vi "_FPGA Check Turbo.vi"(4 "error in":errorcluster, 6 "CheckNow (F)":bool) -> (0 "error out":errorcluster, 2 "SpeedOK":bool)   [LabVIEW 2012]
uses:
  Type/_Pump Parameter.ctl
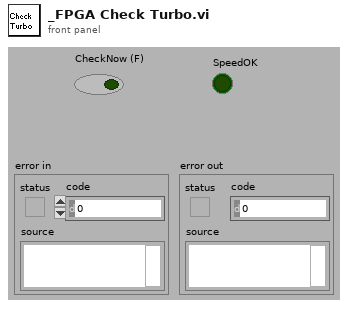
[diagram p1: front panel]
types:
  T1 = typedef "_Pump Parameter.ctl" = enum16{"Turn Pump Motor On", "Turn Pump Motor Off", "Read Pump Oil Deficiency", "Read Rotation Switch Point Attained", "Read Ele. Drive Over Temperature", "Read Pump Over Temperature", "Read Set Rotation Speed Attained", "Read Turbopump Accelerates", "Read Actual Rotation Speed in Hz", "Read Motor Current in A", "Read Operating Hours in h", "Read Motor Voltage in V", "Read Motor Power in W", "Set Rotation Speed Switchpoint in %", "Clear Error", "Read Error Code", "Read Bearing Temperature", "Read Hardware Version", "Read Firmware Version", "Read Operating Hours (Drive)", "Read Rotational Speed (rpm)", "Read Power Stage Temperature", "Read Electronics Temperature", "Read Upper Pump Temperature", "Read Motor Temperature", "Read Error Code History, 1", "Read Error Code History, 2", "Read Error Code History, 3", "Read Error Code History, 4", "Read Error Code History, 5", "Read Error Code History, 6", "Read Error Code History, 7", "Read Error Code History, 8", "Read Error Code History, 9", "Read Error Code History, 10"}
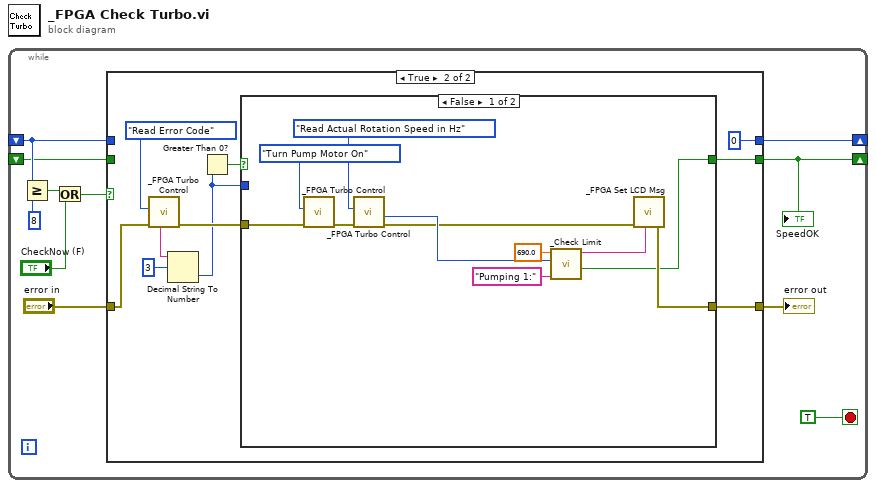
[diagram p0: block diagram]
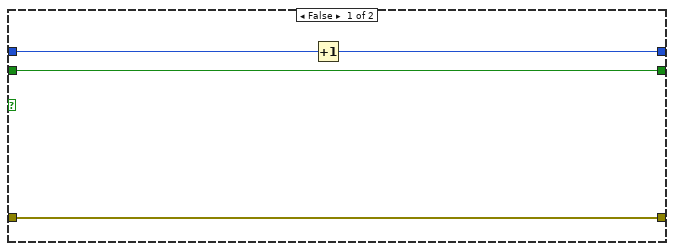
[diagram p2: hidden frame]
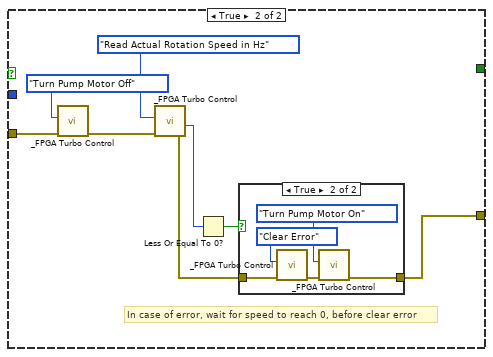
[diagram p3: hidden frame]
diagram:
  n1 = while {
    shift-right: [w10] -> _
    shift-left: _ -> [w5]
    shift-right: [w1] -> _
    shift-left: _ -> [w2]
    stop <- TRUE stop-if-true
    n2 = Greater Or Equal?(x=w5, y=8) -> (x >= y?=w8:bool)
    n3 = Or(x=w8, y="CheckNow (F)") -> (x .or. y?=w6:bool)
    n4 = case shown="True" w6 {
      tunnel: [w14 0] -> w10
      tunnel: w5 -> [w15 _]
      tunnel: [w13 w24] -> w3
      tunnel: "error in" -> [w13 w22]
      tunnel: [w12 w23] -> w1
      tunnel: w2 -> [w12 _]
      frame False {
        n5 = Increment(x=w15) -> (x+1=w14:i32)
      }
      frame True {
        n6 = call "_FPGA Turbo Control.vi"("error in (no error)"=w22, "Command"=_Pump_Parameter."Read Error Code") -> ("error out"=w21:errorcluster, "Error Code"=w18:string)  [unwired: 2 in, 4 out]
        n7 = Decimal String To Number(string=w18, offset=3 ("offset (0)")) -> (number=w16:i32)  [unwired: 2 out]
        n8 = Greater Than 0?(x=w16) -> (x > 0?=w19:bool)
        n9 = case shown="False" w19 {
          tunnel: [w36 w40] -> w24
          tunnel: [w27 _] -> w23
          tunnel: w21 -> [w32 w39]
          tunnel: w16 -> [_ _]
          frame False {
            n10 = call "_FPGA Turbo Control.vi"("error in (no error)"=w32, "Command"=_Pump_Parameter."Turn Pump Motor On") -> ("error out"=w34:errorcluster)  [unwired: 2 in, 5 out]
            n11 = call "_FPGA Turbo Control.vi"("error in (no error)"=w34, "Command"=_Pump_Parameter."Read Actual Rotation Speed in Hz") -> ("error out"=w29:errorcluster, "Speed"=w30:i32)  [unwired: 2 in, 4 out]
            n12 = call "_Check Limit.vi"("Header"="Pumping 1:", "Current"=w30, "Max (100)"=690.0) -> ("Max Reached"=w27:bool, "ProgressBar"=w28:string)  [unwired: 1 in, 2 out]
            n13 = call "_FPGA Set LCD Msg.vi"("Info"=w28, "error in"=w29) -> ("error out"=w36:errorcluster)  [unwired: 5 in, 2 out]
          }
          frame True {
            # "In case of error, wait for speed to reach 0, before clear error"
            n14 = call "_FPGA Turbo Control.vi"("error in (no error)"=w39, "Command"=_Pump_Parameter."Turn Pump Motor Off") -> ("error out"=w38:errorcluster)  [unwired: 2 in, 5 out]
            n15 = call "_FPGA Turbo Control.vi"("error in (no error)"=w38, "Command"=_Pump_Parameter."Read Actual Rotation Speed in Hz") -> ("error out"=w41:errorcluster, "Speed"=w43:i32)  [unwired: 2 in, 4 out]
            n16 = Less Or Equal To 0?(x=w43) -> (x <= 0?=w42:bool)
            n17 = case shown="True" w42 {
              tunnel: w41 -> [w45 w50]
              tunnel: [w45 w46] -> w40
              frame False {
              }
              frame True {
                n18 = call "_FPGA Turbo Control.vi"("error in (no error)"=w50, "Command"=_Pump_Parameter."Clear Error") -> ("error out"=w48:errorcluster)  [unwired: 2 in, 5 out]
                n19 = call "_FPGA Turbo Control.vi"("error in (no error)"=w48, "Command"=_Pump_Parameter."Turn Pump Motor On") -> ("error out"=w46:errorcluster)  [unwired: 2 in, 5 out]
              }
            }
          }
        }
      }
    }
    "error out" <- w3
    "SpeedOK" <- w1
  }
